vi "CMI Sync V3 Set Channel 1 Division Factors.vi"(6 "DDS absolute [Hz] (1 MHz)":dbl=1000000.0, 7 "DDS ratio (1.0)":dbl=1.0, 8 "error in":errorcluster, 9 "DDS multiplier (1)":i32=1, 10 "Divider (10)":i32=10, 11 "session in":T1={"VISA"="", "baud rate [bd/s]"=115200, "source"=enum."Auto", "hv range"=enum."1kV", "fsrc is fixed"=FALSE, "fsrc [Hz]"=10000000.0, "freq integ [s]"=1.0, "freq filter"=5, "trig level"=enum."TTL 5V", "chn1 mode"=enum."Source divider", "chn1 level"=enum."Positive 5V", "chn2 mode"=enum."Source divider", "chn2 level"=enum."Positive 5V", "chn2 div"=1, "chn3 mode"=enum."Chn 1 Active", "chn3 level"=enum."Positive 5V"} {"chn2 div" min=1 max=100000000 step=1; "fsrc [Hz]" format="%_8p"}) -> (0 "error out":errorcluster, 3 "session out":T1={"VISA"="", "baud rate [bd/s]"=115200, "source"=enum."Auto", "hv range"=enum."1kV", "fsrc is fixed"=FALSE, "fsrc [Hz]"=10000000.0, "freq integ [s]"=1.0, "freq filter"=5, "trig level"=enum."TTL 5V", "chn1 mode"=enum."Source divider", "chn1 level"=enum."Positive 5V", "chn2 mode"=enum."Source divider", "chn2 level"=enum."Positive 5V", "chn2 div"=1, "chn3 mode"=enum."Chn 1 Active", "chn3 level"=enum."Positive 5V"} {"chn2 div" min=1 max=100000000 step=1; "fsrc [Hz]" format="%_8p"})   [LabVIEW 2020, in "AWG.lvlib" / "CMI Sync Unit V3.lvlib"]
doc: "Sets output frequency of channel 1 (divisor, multiplier, DDS factor and DDS absolute frequency). Priority/selection of the actual ratio/frequency depends on set mode of the channel."
uses:
  CMI Sync Unit V3.lvlib
  CMI Sync V3 session.ctl
  CMI Sync V3 Reference Clock Source.ctl
  CMI Sync V3 HV input Range.ctl
  CMI Sync V3 Trigger Input Level.ctl
  CMI Sync V3 Channel 1 Mode.ctl
  CMI Sync V3 Channel Output Levels.ctl
  CMI Sync V3 Channel 2 Mode.ctl
  CMI Sync V3 Channel 3 Mode.ctl
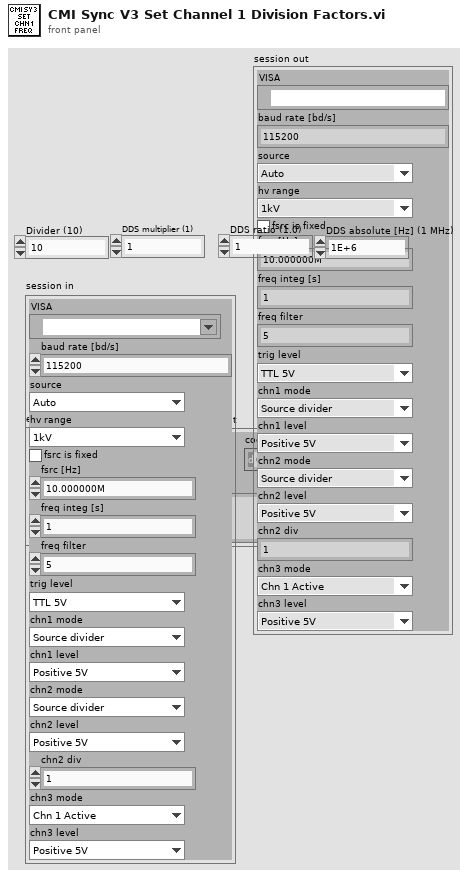
[diagram p1: front panel]
types:
  T1 = typedef "AWG.lvlib/CMI Sync Unit V3.lvlib/CMI Sync V3 session.ctl" = cluster{"VISA":refnum<visa-resource-name>, "baud rate [bd/s]":i32, "source":T2, "hv range":T3, "fsrc is fixed":bool, "fsrc [Hz]":dbl, "freq integ [s]":dbl, "freq filter":i32, "trig level":T4, "chn1 mode":T5, "chn1 level":T6, "chn2 mode":T7, "chn2 level":T6, "chn2 div":i32, "chn3 mode":T8, "chn3 level":T6}
  T2 = typedef "AWG.lvlib/CMI Sync Unit V3.lvlib/CMI Sync V3 Reference Clock Source.ctl" = enum16{"Auto", "Internal", "Logic", "Sine", "HV"}
  T3 = typedef "AWG.lvlib/CMI Sync Unit V3.lvlib/CMI Sync V3 HV input Range.ctl" = enum16{"10V", "60V", "250V", "1kV"}
  T4 = typedef "AWG.lvlib/CMI Sync Unit V3.lvlib/CMI Sync V3 Trigger Input Level.ctl" = enum16{"LVCMOS 3V3", "TTL 5V"}
  T5 = typedef "AWG.lvlib/CMI Sync Unit V3.lvlib/CMI Sync V3 Channel 1 Mode.ctl" = enum16{"Source divider", "DDS absolute", "DDS ratio", "DDS ratio M/N"}
  T6 = typedef "AWG.lvlib/CMI Sync Unit V3.lvlib/CMI Sync V3 Channel Output Levels.ctl" = enum16{"Positive 3V3", "Negative 3V3", "Positive 5V", "Negative 5V"}
  T7 = typedef "AWG.lvlib/CMI Sync Unit V3.lvlib/CMI Sync V3 Channel 2 Mode.ctl" = enum16{"Source divider", "Chn 1 divide"}
  T8 = typedef "AWG.lvlib/CMI Sync Unit V3.lvlib/CMI Sync V3 Channel 3 Mode.ctl" = enum16{"Chn 1 Active", "Chn 2 Active", "Chn 1 Trigger", "Chn 2 Trigger", "Gate", "PPS", "10MHz"}
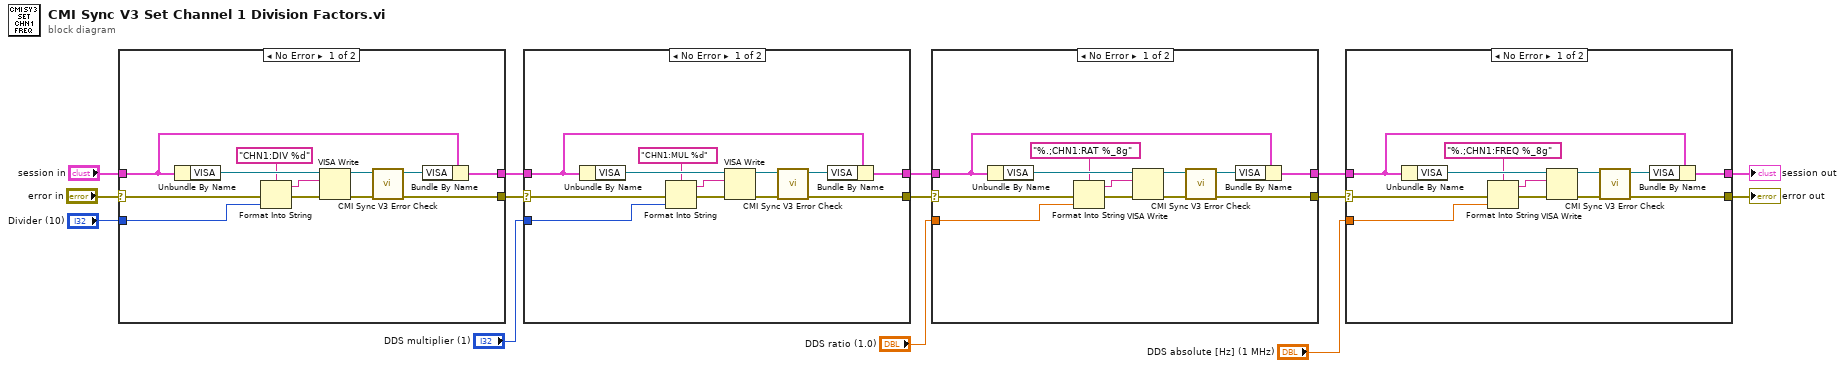
[diagram p0: block diagram]
diagram:
  n1 = case shown="No Error" "error in" {
    selector: "error in" -> [w19 w28]
    tunnel: "session in" -> [w26 w27]
    tunnel: [w25 w27] -> w10
    tunnel: [w20 w28] -> w11
    tunnel: "Divider (10)" -> [w15 _]
    frame No Error {
      n2 = Unbundle By Name(w26) -> ("VISA"=w24:refnum<visa-resource-name>)
      n3 = Format Into String(format string="CHN1:DIV %d", error in=w19, w15) -> (resulting string=w17:string, error out=w18:errorcluster)  [unwired: 1 in]
      n4 = VISA Write(VISA resource name=w24, write buffer=w17, error in (no error)=w18) -> (VISA resource name out=w22:refnum<visa-resource-name>, error out=w23:errorcluster)  [unwired: 1 out]
      n5 = call "CMI Sync V3 Error Check.vi"("error in"=w23, "VISA in"=w22) -> ("error out"=w20:errorcluster, "VISA out"=w21:refnum<visa-resource-name>)  [unwired: 7 in, 1 out]
      n6 = Bundle By Name(cluster=w26, "VISA"=w21) -> (w25:T1)
    }
    frame Error {
    }
  }
  n7 = case shown="No Error" w11 {
    selector: w11 -> [w33 w42]
    tunnel: w10 -> [w40 w41]
    tunnel: [w39 w41] -> w7
    tunnel: [w34 w42] -> w8
    tunnel: "DDS multiplier (1)" -> [w29 _]
    frame No Error {
      n8 = Unbundle By Name(w40) -> ("VISA"=w38:refnum<visa-resource-name>)
      n9 = Format Into String(format string="CHN1:MUL %d", error in=w33, w29) -> (resulting string=w31:string, error out=w32:errorcluster)  [unwired: 1 in]
      n10 = VISA Write(VISA resource name=w38, write buffer=w31, error in (no error)=w32) -> (VISA resource name out=w36:refnum<visa-resource-name>, error out=w37:errorcluster)  [unwired: 1 out]
      n11 = call "CMI Sync V3 Error Check.vi"("error in"=w37, "VISA in"=w36) -> ("error out"=w34:errorcluster, "VISA out"=w35:refnum<visa-resource-name>)  [unwired: 7 in, 1 out]
      n12 = Bundle By Name(cluster=w40, "VISA"=w35) -> (w39:T1)
    }
    frame Error {
    }
  }
  n13 = case shown="No Error" w8 {
    selector: w8 -> [w47 w56]
    tunnel: w7 -> [w54 w55]
    tunnel: [w53 w55] -> w4
    tunnel: [w48 w56] -> w5
    tunnel: "DDS ratio (1.0)" -> [w43 _]
    frame No Error {
      n14 = Unbundle By Name(w54) -> ("VISA"=w52:refnum<visa-resource-name>)
      n15 = Format Into String(format string="%.;CHN1:RAT %_8g", error in=w47, w43) -> (resulting string=w45:string, error out=w46:errorcluster)  [unwired: 1 in]
      n16 = VISA Write(VISA resource name=w52, write buffer=w45, error in (no error)=w46) -> (VISA resource name out=w50:refnum<visa-resource-name>, error out=w51:errorcluster)  [unwired: 1 out]
      n17 = call "CMI Sync V3 Error Check.vi"("error in"=w51, "VISA in"=w50) -> ("error out"=w48:errorcluster, "VISA out"=w49:refnum<visa-resource-name>)  [unwired: 7 in, 1 out]
      n18 = Bundle By Name(cluster=w54, "VISA"=w49) -> (w53:T1)
    }
    frame Error {
    }
  }
  n19 = case shown="No Error" w5 {
    selector: w5 -> [w61 w70]
    tunnel: w4 -> [w68 w69]
    tunnel: [w67 w69] -> w2
    tunnel: [w62 w70] -> w1
    tunnel: "DDS absolute [Hz] (1 MHz)" -> [w57 _]
    frame No Error {
      n20 = Unbundle By Name(w68) -> ("VISA"=w66:refnum<visa-resource-name>)
      n21 = Format Into String(format string="%.;CHN1:FREQ %_8g", error in=w61, w57) -> (resulting string=w59:string, error out=w60:errorcluster)  [unwired: 1 in]
      n22 = VISA Write(VISA resource name=w66, write buffer=w59, error in (no error)=w60) -> (VISA resource name out=w64:refnum<visa-resource-name>, error out=w65:errorcluster)  [unwired: 1 out]
      n23 = call "CMI Sync V3 Error Check.vi"("error in"=w65, "VISA in"=w64) -> ("error out"=w62:errorcluster, "VISA out"=w63:refnum<visa-resource-name>)  [unwired: 7 in, 1 out]
      n24 = Bundle By Name(cluster=w68, "VISA"=w63) -> (w67:T1)
    }
    frame Error {
    }
  }
  "error out" <- w1
  "session out" <- w2
